vi "OE1201_Query Data.vi"(0 "VISA resource name":refnum<visa-resource-name>, 9 "Remote Mode":u16(ring) items=["USB", "RS232"], 11 "Error in (no error)":errorcluster caption="error out（no error）") -> (4 "VISA resource  out":refnum<visa-resource-name>, 6 "Parameter Values":T1={"R"=0.1, "X"=0.1, "Y"=0.1, "θ"=0.1, "Freq"=0.1} {"Freq" min=0.1 max=1.0 format="%.6f"; "θ" min=0.1 max=1.0 format="%.6f"; "Y" min=0.1 max=1.0 format="%.6f"; "X" min=0.1 max=1.0 format="%.6f"; "R" min=0.1 max=1.0 format="%.6f"}, 8 "Data Array":dbl[](array[numeric]), 10 "Output String":string, 15 "Error out":errorcluster caption="error out")   [LabVIEW 2011]
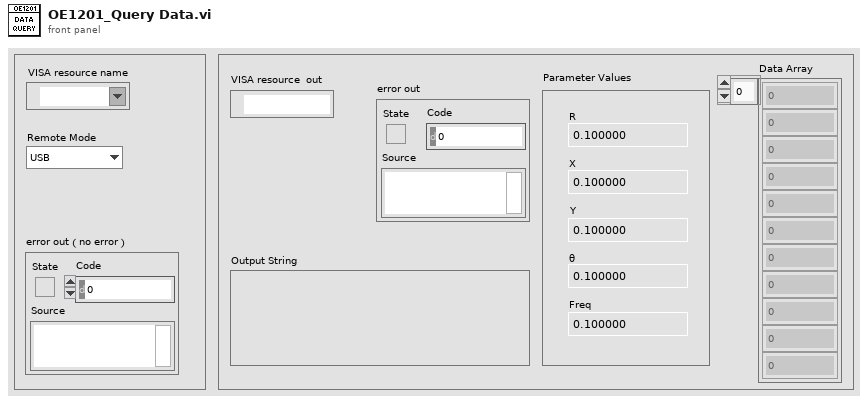
[diagram p1: front panel]
types:
  T1 = cluster{"R":dbl, "X":dbl, "Y":dbl, "θ":dbl, "Freq":dbl}
  T2 = enum16{"ISRC", "IGND", "ICPL", "ILIN", "PHAS", "FMOD", "RSLP", "FREQ", "SWPT", "SLLM", "SULM", "SSLL", "SSLG", "STLM", "SWRM", "IRNG", "SENS", "RMOD", "OFLT", "OFSL", "SYNC", "DMOD", "HARM", "DARB", "SWVT", "SLVL", "SVLL", "SVUL", "SVSL", "SVSG", "SVTM", "SVRM", "RALL", "SNAP", "OUTP", "OAUX", "COUT", "CAUX", "COFP", "CEXP", "FPOP", "OEXP", "*IDN", "*RST", "OVLD", "INOV", "GNOV", "*PLL", "SSET", "RSET", "AGAN", "APHS", "ARSV", "ASCL", "EQCD", "EQCS", "SPED", "SRAT", "SLEN", "SSLE", "STRG", "SPRM", "STRD", "PAUS", "REST", "SPTS", "TRCA", "TEMP", "RSTU", "IHNZ", "DEQU", "SADD", "ARNG", "CSPE", "ISRCD", "IGNDD", "ICPLD", "ILIND", "PHASD", "FMODD", "RSLPD", "FREQD", "SWPTD", "SLLMD", "SULMD", "SSLLD", "SSLGD", "STLMD", "SWRMD", "SENSD", "RMODD", "OFLTD", "OFSLD", "SYNCD", "HARMD", "EQCDD", "EQCSD", "SNAPD", "OUTPD", "SWVTD", "SLVLD", "SVLLD", "SVULD", "SVSLD", "SVSGD", "SVTMD", "SVRMD", "SVDCD", "ARSVD", "AGAND", "APHSD", "ASCLD", "FPOPD", "CAUXD", "OEXPD", "SPEDD", "SRATD", "SLEND", "SSLED", "STRGD", "SPRMD", "STRDD", "PAUSD", "RESTD", "SPTSD", "TRCAD", "*IDND", "*RSTD", "INOVD", "GNOVD", "*PLLD", "SSETD", "RSETD"}
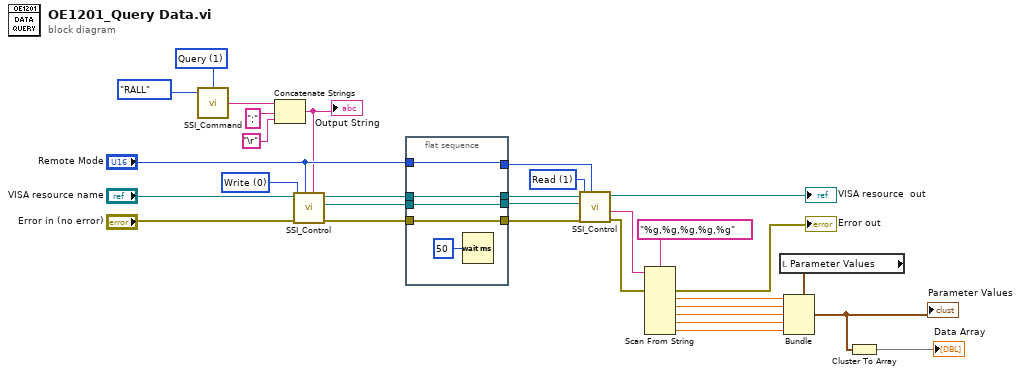
[diagram p0: block diagram]
diagram:
  w15 = u16 1 items=["Write", "Read"] ("Control")
  w23 = u16 1 items=["Set", "Query"] ("Opera")
  w27 = u16 0 items=["Write", "Read"] ("Control")
  n1 = call "SSI_Command.vi"("Opera"=w23, "Command Type"=T2."RALL") -> ("Output string"=w24:string)  [unwired: 2 in]
  n2 = Concatenate Strings(w24, ";" ("替换字符串(\"\")"), "\r") -> (w13:string)
  "Output String" <- w13
  n3 = call "SSI_Control.vi"("Write Buffer"=w13, "Remote Mode"="Remote Mode", "Error in (no error)"="Error in (no error)", "Control"=w27, "VISA resource name"="VISA resource name") -> ("Error out"=w20:errorcluster, "Connection ID out"=w17:refnum<k5>, "VISA resource  out"=w21:refnum<visa-resource-name>)  [unwired: 3 in, 1 out]
  n4 = flat-sequence {
    tunnel: w21 -> [w36]
    tunnel: w20 -> [w35]
    tunnel: [w36] -> w19
    tunnel: [w35] -> w18
    tunnel: [w33] -> w16
    tunnel: w17 -> [w33]
    tunnel: [w32] -> w14
    tunnel: "Remote Mode" -> [w32]
    frame #0 {
      n5 = Wait (ms)(milliseconds to wait=u32 50 ("等待时间（毫秒）")) -> ()  [unwired: 1 out]
    }
  }
  n6 = call "SSI_Control.vi"("Remote Mode"=w14, "Error in (no error)"=w18, "Control"=w15, "Connection ID in"=w16, "VISA resource name"=w19) -> ("Error out"=w11:errorcluster, "Read Buffer"=w12:string, "VISA resource  out"=→"VISA resource  out":refnum<visa-resource-name>)  [unwired: 3 in, 1 out]
  n7 = Scan From String(format string="%g,%g,%g,%g,%g" ("格式字符串"), input string=w12, error in=w11) -> (error out=→"Error out":errorcluster, output 1=w9:dbl, output 2=w8:dbl, output 3=w7:dbl, output 4=w6:dbl, output 5=w5:dbl)  [unwired: 6 in, 2 out]
  n8 = local read "Parameter Values"() -> (w3:T1)
  n9 = Bundle(cluster=w3, "R"=w9, "X"=w8, "Y"=w7, "θ"=w6, "Freq"=w5) -> (w2:T1)
  "Parameter Values" <- w2
  n10 = Cluster To Array(cluster=w2) -> (array=→"Data Array":dbl[])
